vi "Fetch Measurement (Data Rate-Unit Interval).vi"(0 "VISA resource name":refnum<visa-resource-name>, 5 "Channel (1: Channel 1)":i32(ring)=1 items=["Channel 1"=1, "Channel 2"=2, "Channel 3"=3, "Channel 4"=4, "Function 1"=5, "Function 2"=6, "Function 3"=7, "Function 4"=8, "Memory 1"=9, "Memory 2"=10, "Memory 3"=11, "Memory 4"=12], 7 "Measurement (0: Data Rate)":i32(ring) items=["Data Rate", "Unit Interval"], 9 "Data Rate Type (0: Fully Automatic)":i32(ring) items=["Fully Automatic", "Semi Automatic"], 11 "error in (no error)":errorcluster, 12 "Data Rate (2.5E9 Hz)":dbl=2500000000.0) -> (4 "VISA resource name out":refnum<visa-resource-name>, 6 "Measurement":dbl, 15 "error out":errorcluster)   [LabVIEW 2012, in "Agilent 8000 Series.lvlib"]
doc: "Returns the results of the Data Rate or Unit Interval measurement."
uses:
  Agilent 8000 Series.lvlib
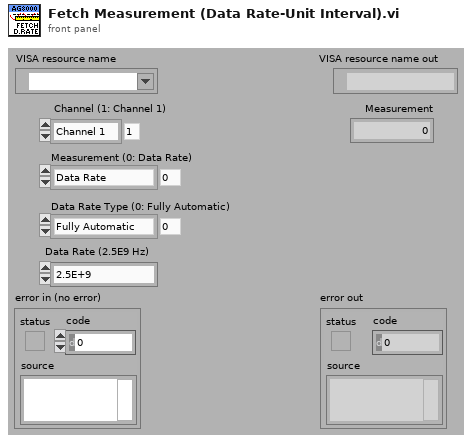
[diagram p1: front panel]
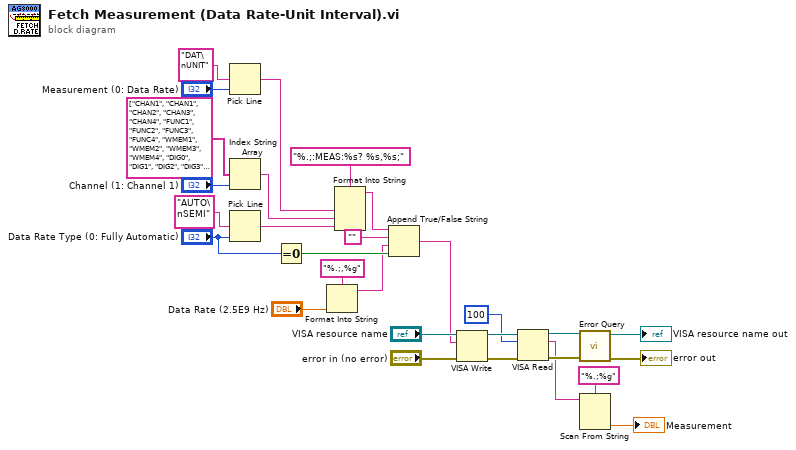
[diagram p0: block diagram]
diagram:
  n1 = Pick Line(multi-line string="DAT\nUNIT", line index="Measurement (0: Data Rate)") -> (output string=w1:string)  [unwired: 1 in]
  n2 = Index String Array(1:"Channel (1: Channel 1)", 2:string[] ["CHAN1", "CHAN1", "CHAN2", "CHAN3", "CHAN4", "FUNC1", "FUNC2", "FUNC3", "FUNC4", "WMEM1", "WMEM2", "WMEM3", "WMEM4", "DIG0", "DIG1", "DIG2", "DIG3", "DIG4", "DIG5", "DIG6", "DIG7", "DIG8", "DIG9", "DIG10", "DIG11", "DIG12", "DIG13", "DIG14", "DIG15", "AUX", "LINE"]) -> (0:w2:string)  [unwired: 1 in]
  n3 = Pick Line(multi-line string="AUTO\nSEMI", line index="Data Rate Type (0: Fully Automatic)") -> (output string=w3:string)  [unwired: 1 in]
  n4 = Equal To 0?(x="Data Rate Type (0: Fully Automatic)") -> (x = 0?=w20:bool)
  n5 = Format Into String(format string="%.;,%g", "Data Rate (2.5E9 Hz)") -> (resulting string=w16:string)  [unwired: 2 in, 1 out]
  n6 = Format Into String(format string="%.;:MEAS:%s? %s,%s;", w1, w2, w3) -> (resulting string=w15:string)  [unwired: 2 in, 1 out]
  n7 = Append True/False String(1:w20, 2:w16, 3:"", 4:w15) -> (0:w14:string)
  n8 = VISA Write(VISA resource name="VISA resource name", write buffer=w14, error in (no error)="error in (no error)") -> (VISA resource name out=w12:refnum<visa-resource-name>, error out=w13:errorcluster)  [unwired: 1 out]
  n9 = VISA Read(VISA resource name=w12, byte count=u32 100, error in (no error)=w13) -> (VISA resource name out=w11:refnum<visa-resource-name>, read buffer=w8:string, error out=w9:errorcluster)  [unwired: 1 out]
  n10 = call "Error Query.vi"("error in (no error)"=w9, "VISA resource name"=w11) -> ("error out"=→"error out":errorcluster, "VISA resource name out"=→"VISA resource name out":refnum<visa-resource-name>)  [unwired: 6 in, 2 out]
  n11 = Scan From String(format string="%.;%g", input string=w8) -> (output 1=→"Measurement":dbl)  [unwired: 3 in, 3 out]
